vi "PM_FPGA.vi"() -> ()   [LabVIEW 2019]
uses:
  <vilib>/rvi/Emulation/niFpgaGetClockAttributes.vi
  <vilib>/rvi/Emulation/niFpgaSctlEmulationGetInTimedLoop.vi
  <vilib>/rvi/Emulation/niFpgaEmulationReportErrorSimple.vi
  <vilib>/rvi/eio/common/nirviEmuTemplateMethod_errors.vi
  <vilib>/rvi/Emulation/niFpgaCriticalErrorInLSC.vi
  <vilib>/rvi/Emulation/niFpgaProcessEmulError.vi
  <vilib>/eio/EIONode/EIONode.xnode
panel:
  in  "Cam":bool
  out "cam report":bool
  in  "trigger":bool
  in  "stop":bool
  out "volt":i16
  out "Count":u32 caption="Tick Count(uSec)"
  out "Load":u16
  in  "Count(uSec)":u32
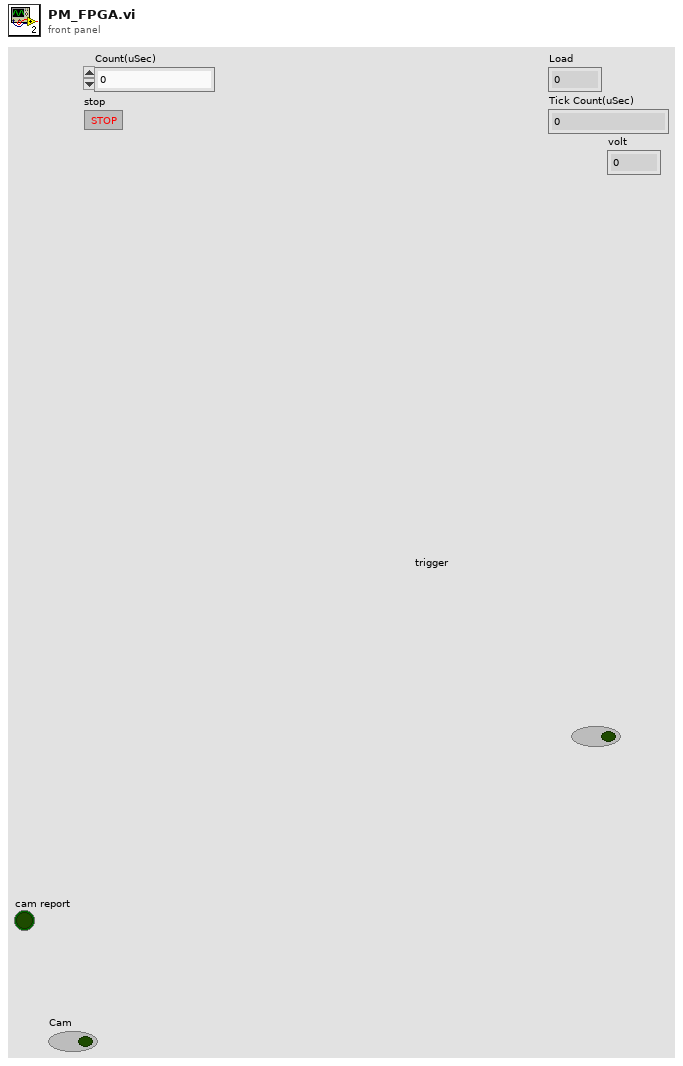
[diagram p1: front panel]
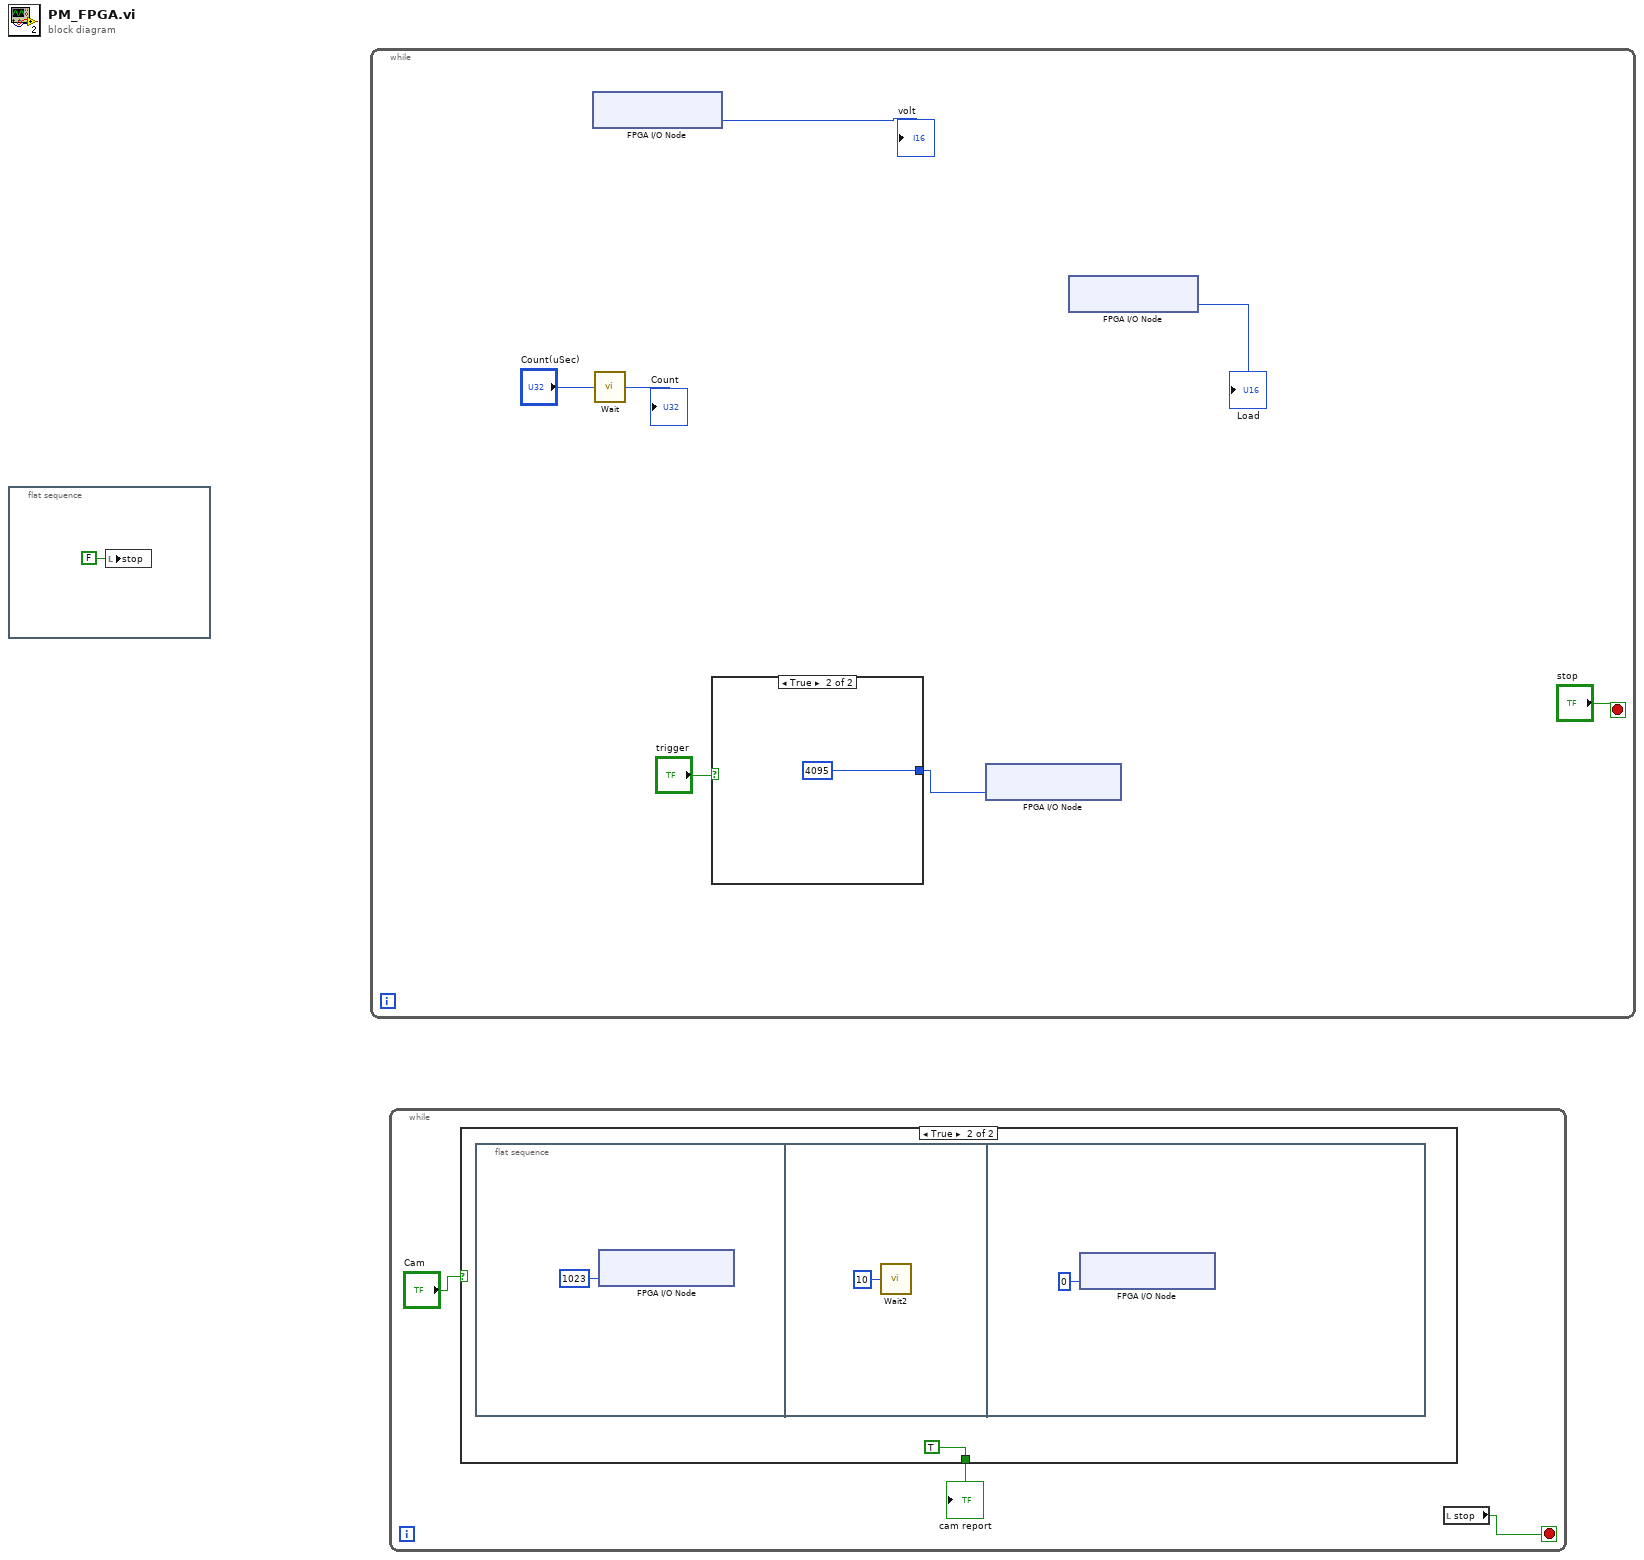
[diagram p0: block diagram]
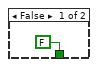
[diagram p2: hidden frame]
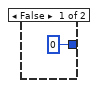
[diagram p3: hidden frame]
diagram:
  n1 = flat-sequence {
    frame #0 {
      n2 = local write "stop"(FALSE ("stop")) -> ()
    }
  }
  n3 = while {
    stop <- "stop" stop-if-true
    n4 = xnode "FPGA I/O Node"() -> ("ConnectorC/AI0"=→"volt":i16)  [unwired: 1 in, 1 out]
    n5 = call "Wait"("Count(uSec)"="Count(uSec)") -> ("Tick Count(uSec)"=→"Count":u32)
    n6 = case shown="True" "trigger" {
      tunnel: [u16 0 ("ConnectorA/AO0") u16 4095 ("ConnectorA/AO0")] -> w3
      frame False {
      }
      frame True {
      }
    }
    n7 = xnode "FPGA I/O Node"("ConnectorA/AO0"=w3) -> ()  [unwired: 1 in, 1 out]
    n8 = xnode "FPGA I/O Node"() -> ("ConnectorA/AI1"=→"Load":u16)  [unwired: 1 in, 1 out]
  }
  n9 = while {
    stop <- w12 stop-if-true
    n10 = case shown="True" "Cam" {
      tunnel: [FALSE TRUE] -> w11
      frame False {
      }
      frame True {
        n11 = flat-sequence {
          frame #0 {
            n12 = xnode "FPGA I/O Node"("ConnectorC/AO0"=i16 1023) -> ()  [unwired: 1 in, 1 out]
          }
          frame #1 {
            n13 = call "Wait2"("Count(mSec)"=u32 10) -> ()  [unwired: 1 out]
          }
          frame #2 {
            n14 = xnode "FPGA I/O Node"("ConnectorC/AO0"=i16 0) -> ()  [unwired: 1 in, 1 out]
          }
        }
      }
    }
    "cam report" <- w11
    n15 = local read "stop"() -> (w12:bool)
  }
